vi "pnumatics Controller.vi"(8 "error in":errorcluster) -> ()   [LabVIEW 2015]
doc: "This VI executes continuously carrying out the current operation and responding to updates or new operations. It will often contain the timing or control code that is difficult to place directly in TeleOp. This VI generally opens all sensors and motors and isolates the rest of the robot code from knowing how the operations are carried out."
uses:
  pnumatics Setpoints.ctl
  pnumatics Operations.ctl
  <vilib>/Rock Robotics/WPI/Solenoid/WPI_SolenoidValue.ctl
  <vilib>/Rock Robotics/Network Tables/NT Write Boolean.vi
panel:
  out "Current\nCmd":string
  # "Tip: It may be helpful to observe inputs and sensor values.\nYou may also want to display tuning or debugging controls."
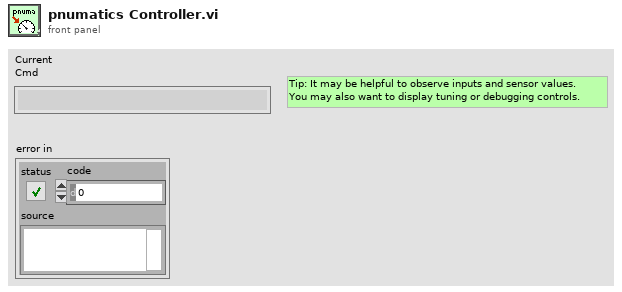
[diagram p1: front panel]
types:
  T1 = typedef "pnumatics Setpoints.ctl" = cluster{"Operation":T2, "Setpoint":dbl, "Duration":dbl, "Intake":dbl}
  T2 = typedef "pnumatics Operations.ctl" = enum16{"Reserve", "Read Current", "Immediate"}
  T3 = typedef "Command Status Info.ctl" = cluster{"Name":string, "Status":T4, "notifier out":T5}
  T4 = typedef "Completion Status.ctl" = enum16{"Successful", "Aborted", "Incomplete"}
  T5 = typedef "Completion Notifier.ctl" = refnum<notifier>
  T6 = cluster{"Default Command":T1, "Command Timing":cluster{"Start Time (ms)":u32, "Iterations":i32}, "Command Arguments":cluster{"Command Info":T3, "Description":string, "Default Command":T1, "notifier out":refnum<notifier>, "Subsystem Name":string}}
  T7 = typedef "WPI_SolenoidValue.ctl" = enum16{"Off", "On", "Forward", "Reverse"}
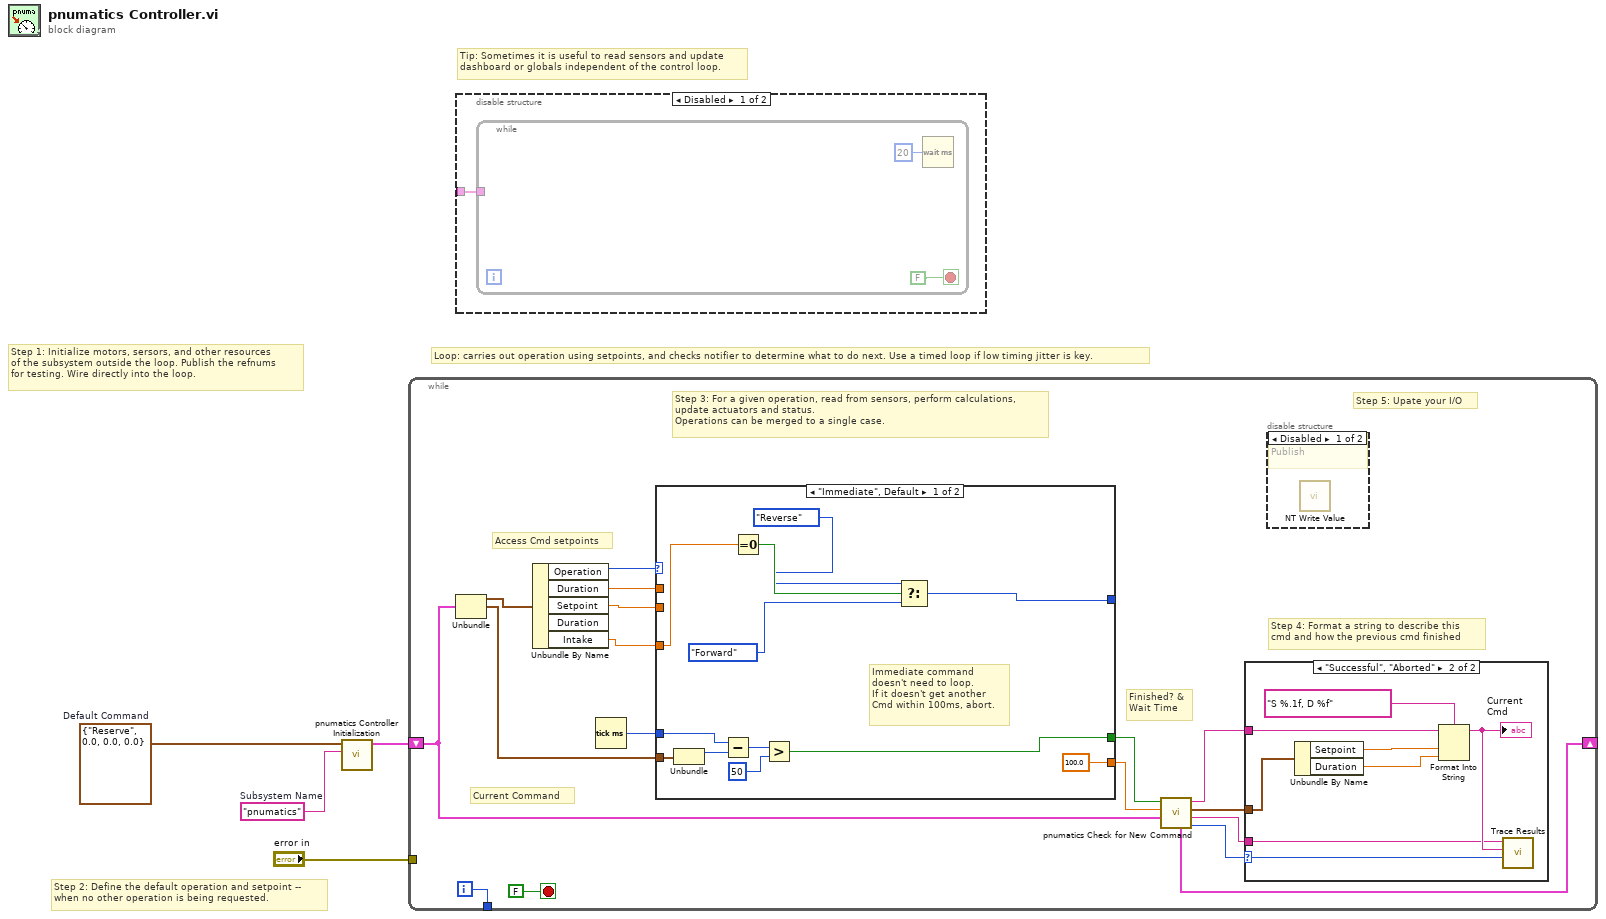
[diagram p0: block diagram]
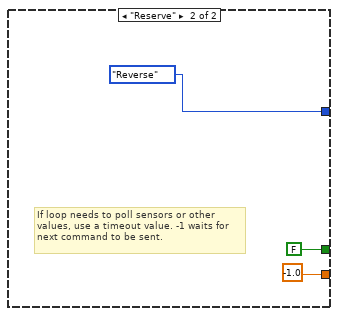
[diagram p5: hidden frame]
diagram:
  w1 = T1 {"Operation"=enum."Reserve", "Setpoint"=0.0, "Duration"=0.0, "Intake"=0.0}  # Default Command
  w2 = "pnumatics"  # Subsystem Name
  # "Tip: Sometimes it is useful to read sensors and update\ndashboard or globals independent of the control loop."
  # "Step 2: Define the default operation and setpoint --\nwhen no other operation is being requested."
  # "Step 1: Initialize motors, sersors, and other resources\nof the subsystem outside the loop. Publish the refnums\nfor testing. Wire directly into the loop."
  # "Loop: carries out operation using setpoints, and checks notifier to determine what to do next. Use a timed loop if low timing jitter is key."
  n1 = call "pnumatics Controller Initialization.vi"("Subsystem Name"=w2, "Default Command"=w1) -> ("Command Info"=w3:T6)  [unwired: 9 in]
  n2 = while {
    shift-right: [w12] -> _
    shift-left: w3 -> [w13]
    tunnel: [w20] -> _
    tunnel: "error in" -> [_]
    i -> [w20]
    stop <- FALSE stop-if-true
    # "Step 5: Upate your I/O"
    # "Step 4: Format a string to describe this\ncmd and how the previous cmd finished"
    # "Current Command"
    # "Access Cmd setpoints"
    # "Finished? &\nWait Time"
    # "Step 3: For a given operation, read from sensors, perform calculations,\nupdate actuators and status.\nOperations can be merged to a single case."
    n3 = Unbundle(w13) -> ("Default Command"=w19:T1, "Command Timing"=w15:cluster{"Start Time (ms)":u32, "Iterations":i32})  [unwired: 1 out]
    n4 = Unbundle By Name(w19) -> ("Operation"=w18:T2, "Duration"=w17:dbl, "Setpoint"=w14:dbl, "Intake"=w5:dbl)  [unwired: 1 out]
    n5 = Tick Count (ms)() -> (millisecond timer value=w16:u32)
    n6 = case shown="\"Immediate\", Default" w18 {
      tunnel: [100.0 -1.0] -> w10
      tunnel: [w35 FALSE ("ignore previous (F)")] -> w11
      tunnel: w15 -> [w37 _]
      tunnel: w17 -> [_ _]
      tunnel: w16 -> [w36 _]
      tunnel: w14 -> [_ _]
      tunnel: w5 -> [w34 _]
      tunnel: [w30 WPI_SolenoidValue."Reverse" ("Value")] -> _
      frame "Immediate", Default {
        # "Immediate command\ndoesn't need to loop.\nIf it doesn't get another\nCmd within 100ms, abort."
        n7 = Unbundle(w37) -> ("Start Time (ms)"=w40:u32)  [unwired: 1 out]
        n8 = Subtract(x=w36, y=w40) -> (x-y=w39:u32)
        n9 = Equal To 0?(x=w34) -> (x = 0?=w33:bool)
        n10 = Greater?(x=w39, y=u8 50 ("Left Motor")) -> (0:w35:bool)
        n11 = Select(t=WPI_SolenoidValue."Reverse" ("Value"), s=w33, f=WPI_SolenoidValue."Forward" ("Value")) -> (s? t:f=w30:T7)
      }
      frame "Reserve" {
        # "If loop needs to poll sensors or other\nvalues, use a timeout value. -1 waits for\nnext command to be sent."
      }
    }
    n12 = call "pnumatics Check for New Command.vi"("Current Command"=w13, "Wait time (ms)"=w10, "Finished?"=w11) -> ("Completion"=w6:T4, "Subsystem Name"=w7:string, "Current Command"=w8:T1, "Initial Trace String"=w9:string, "NextCommand"=w12:T6)  [unwired: 4 in]
    n13 = case shown="\"Successful\", \"Aborted\"" w6 {
      selector: w6 -> [_ w29]
      tunnel: w9 -> [_ w25]
      tunnel: w8 -> [_ w26]
      tunnel: w7 -> [_ w22]
      frame "Incomplete", Default {
        # "Continuing current command"
      }
      frame "Successful", "Aborted" {
        # "Report and setup for next command"
        n14 = Unbundle By Name(w26) -> ("Setpoint"=w28:dbl, "Duration"=w23:dbl)
        n15 = Format Into String(format string="S %.1f, D %f", initial string=w25, w28, w23) -> (resulting string=w24:string)  [unwired: 1 in, 1 out]
        "Current\nCmd" <- w24
        n16 = call <vilib>:"Trace Results.vi"("Status of previous command"=w29, "Description"=w24, "Subsystem"=w22) -> ()  [unwired: 9 in]
      }
    }
    n17 = disable-structure shown="Disabled" {
      frame Disabled {
        # "Publish"
        n18 = call-poly <vilib>:"NT Write Value.vi"() -> ()  [unwired: 11 in, 1 out]
      }
      frame Enabled {
      }
    }
  }
  n19 = disable-structure shown="Disabled" {
    disable-tunnel: _ -> [w45 _]
    frame Disabled {
      n20 = while {
        tunnel: w45 -> [_]
        stop <- FALSE stop-if-true
        n21 = Wait (ms)(milliseconds to wait=u32 20) -> ()  [unwired: 1 out]
      }
    }
    frame Enabled {
    }
  }
